vi "oldVisionToGame.vi"(8 "error in (no error)":errorcluster, 10 "Frame and Field Size in":T5 {"Detection Frame Out"."robots_blue"."height" format="%+4.3f"; "Detection Frame Out"."robots_blue"."pixel_y" format="%+4.3f"; "Detection Frame Out"."robots_blue"."pixel_x" format="%+4.3f"; "Detection Frame Out"."robots_blue"."orientation" format="%+4.3f"; "Detection Frame Out"."robots_blue"."y" format="%+4.3f"; "Detection Frame Out"."robots_blue"."confidence" format="%4.3f"; "Detection Frame Out"."robots_blue"."x" format="%+4.3f"; "Detection Frame Out"."robots_yellow"."height" format="%+4.3f"; "Detection Frame Out"."robots_yellow"."pixel_y" format="%+4.3f"; "Detection Frame Out"."robots_yellow"."pixel_x" format="%+4.3f"; "Detection Frame Out"."robots_yellow"."orientation" format="%+4.3f"; "Detection Frame Out"."robots_yellow"."y" format="%+4.3f"; "Detection Frame Out"."robots_yellow"."confidence" format="%4.3f"; "Detection Frame Out"."robots_yellow"."x" format="%+4.3f"}, 11 "Vision in":refnum<class "Vision.lvclass">) -> (0 "error out":errorcluster, 2 "Detection Frame Out":T1 {"robots_blue"."height" format="%+4.3f"; "robots_blue"."pixel_y" format="%+4.3f"; "robots_blue"."pixel_x" format="%+4.3f"; "robots_blue"."orientation" format="%+4.3f"; "robots_blue"."y" format="%+4.3f"; "robots_blue"."confidence" format="%4.3f"; "robots_blue"."x" format="%+4.3f"; "robots_yellow"."height" format="%+4.3f"; "robots_yellow"."pixel_y" format="%+4.3f"; "robots_yellow"."pixel_x" format="%+4.3f"; "robots_yellow"."orientation" format="%+4.3f"; "robots_yellow"."y" format="%+4.3f"; "robots_yellow"."confidence" format="%4.3f"; "robots_yellow"."x" format="%+4.3f"}, 3 "Vision out":refnum<class "Vision.lvclass">)   [LabVIEW 2022 SP3, in "Vision.lvclass"]
uses:
  Vision.lvclass
  Old vision/Controls/SSL Field State.ctl
  Old vision/Controls/SSL Detection Frame.ctl
  Old vision/Controls/SSL Detection Robot.ctl
  <vilib>/Analysis/Matrix/Datatypes/RealMatrix.ctl
  Old vision/Controls/SSL Detection Ball.ctl
  <vilib>/Analysis/Matrix/NI_Matrix.lvlib
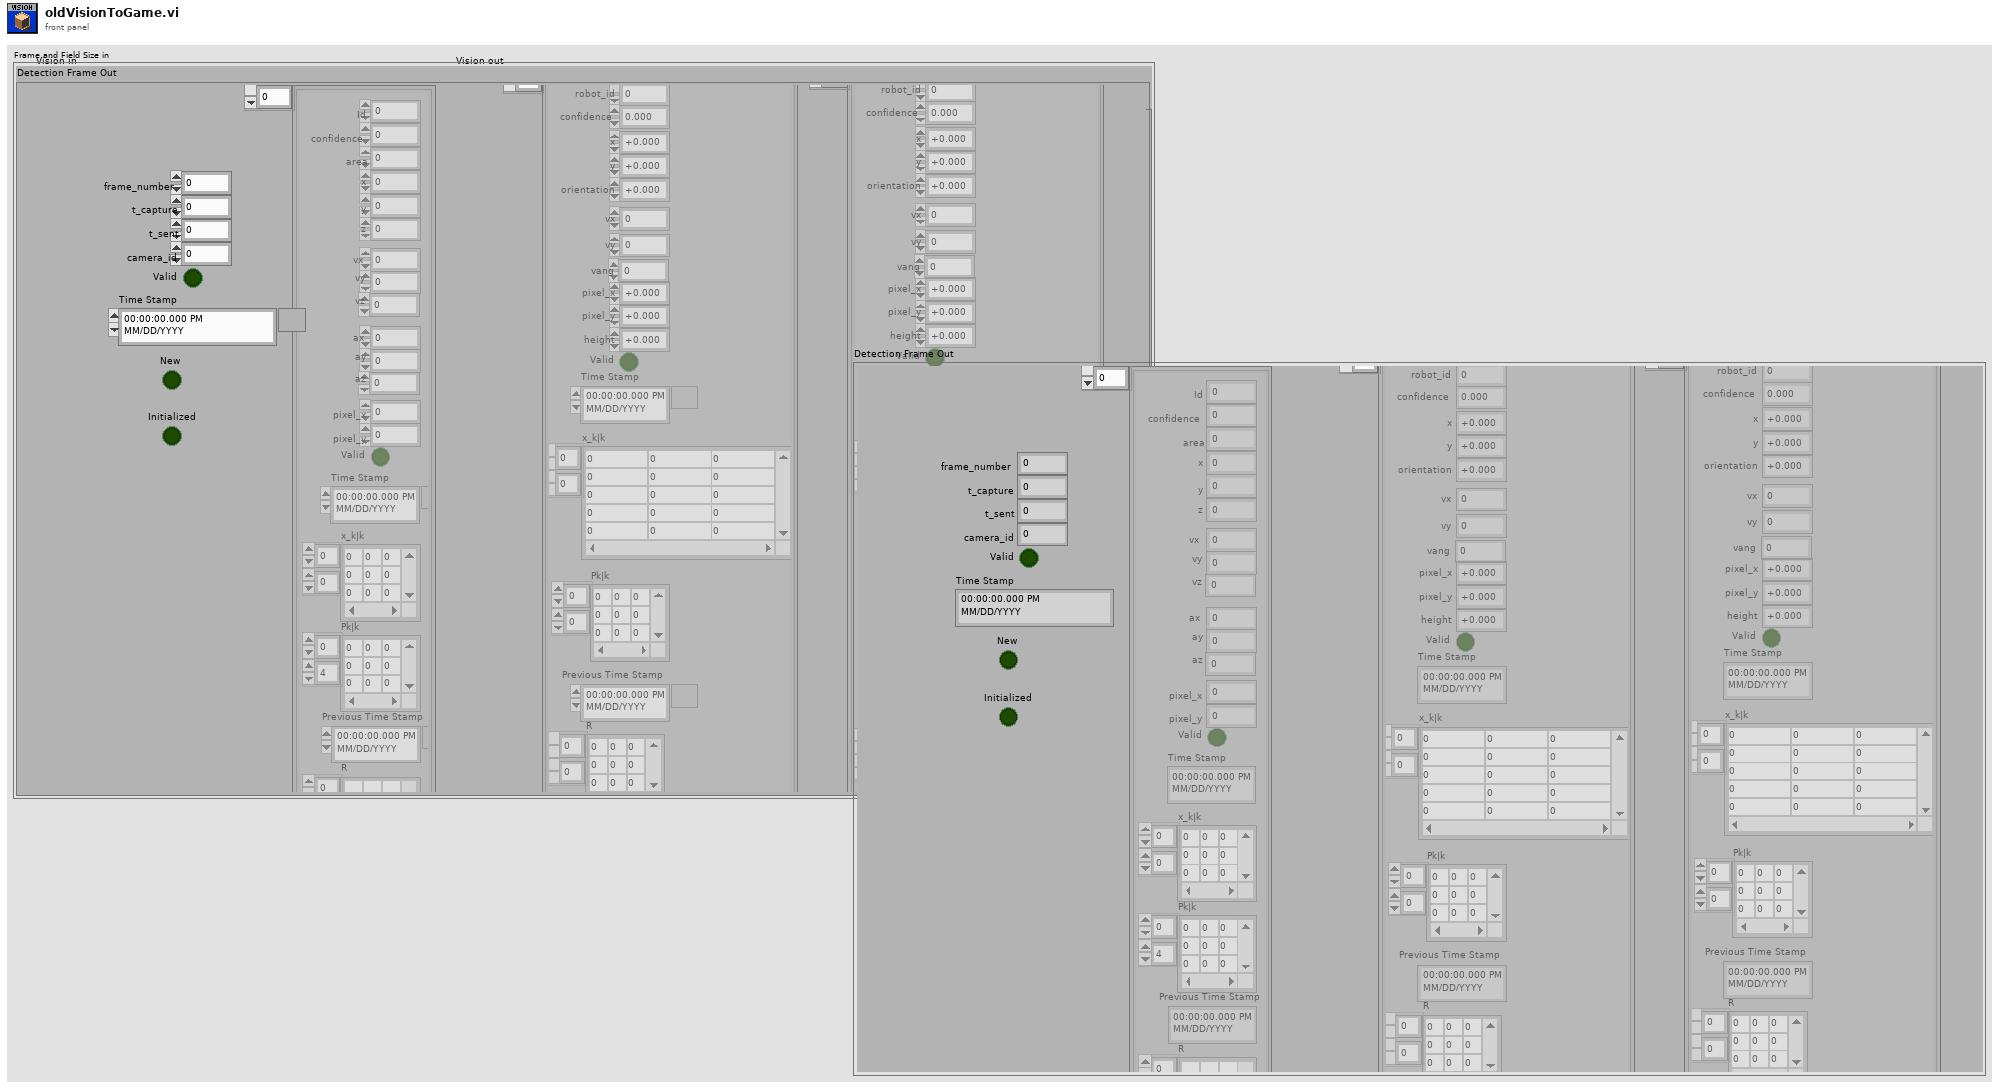
[diagram p1: front panel]
types:
  T1 = typedef "SSL Detection Frame.ctl" = cluster{"frame_number":u32, "t_capture":dbl, "t_sent":dbl, "camera_id":u32, "robots_yellow":T2[], "robots_blue":T2[], "balls":T4[], "Valid":bool, "Time Stamp":timestamp, "New":bool, "Initialized":bool}
  T2 = typedef "SSL Detection Robot.ctl" = cluster{"x":sgl, "robot_id":u32, "confidence":sgl, "y":sgl, "orientation":sgl, "pixel_x":sgl, "pixel_y":sgl, "height":sgl, "Valid":bool, "Time Stamp":timestamp, "x_k|k":T3, "Pk|k":T3, "Previous Time Stamp":timestamp, "R":T3, "vx":dbl, "vy":dbl, "vang":dbl}
  T3 = typedef "NI_Matrix.lvlib/RealMatrix.ctl" = dbl[][]
  T4 = typedef "SSL Detection Ball.ctl" = cluster{"x":sgl, "area":u32, "confidence":sgl, "y":sgl, "z":sgl, "pixel_x":sgl, "pixel_y":sgl, "Valid":bool, "Time Stamp":timestamp, "x_k|k":T3, "Pk|k":T3, "Id":u32, "Previous Time Stamp":timestamp, "R":T3, " vx":sgl, "vy":dbl, "vz":dbl, " ax":sgl, "ay":dbl, "az":dbl}
  T5 = typedef "SSL Field State.ctl" = cluster{"Detection Frame Out":T1, "Field Size Out":cluster{"line_width":u32, "field_length":u32, "field_width":u32, "boundary_width":u32, "referee_width":u32, "goal_width":u32, "goal_depth":u32, "goal_wall_width":u32, "center_circle_radius":u32, "defense_radius":u32, "defense_stretch":u32, "free_kick_from_defense_dist":u32, "penalty_spot_from_field_line_dist":u32, "penalty_line_from_spot_dist":u32}, "Received Time Stamp":timestamp}
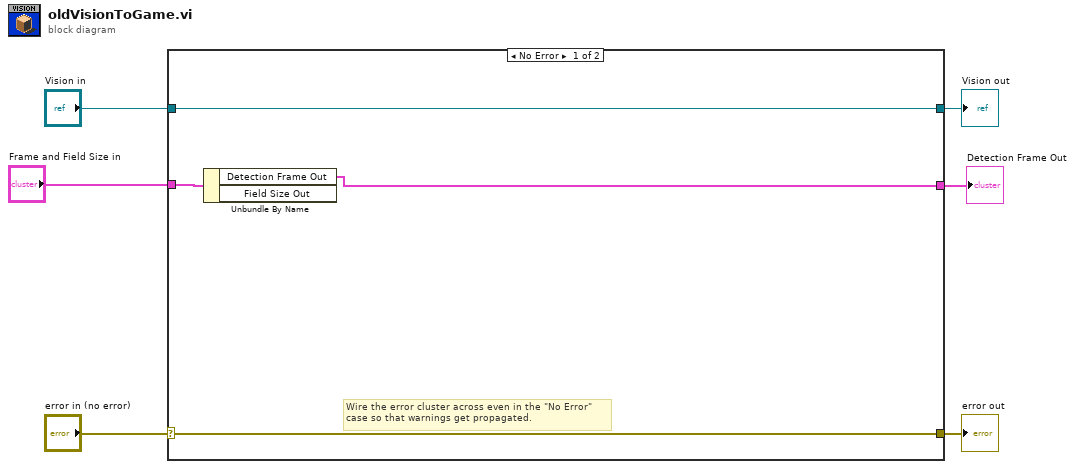
[diagram p0: block diagram]
diagram:
  n1 = case shown="No Error" "error in (no error)" {
    selector: "error in (no error)" -> [w9 w12]
    tunnel: [w9 w12] -> w5
    tunnel: [w10 w11] -> w3
    tunnel: "Vision in" -> [w10 w11]
    tunnel: "Frame and Field Size in" -> [w8 _]
    tunnel: [w7 _] -> w1
    frame No Error {
      # "Wire the error cluster across even in the \"No Error\"\ncase so that warnings get propagated."
      n2 = Unbundle By Name(w8) -> ("Detection Frame Out"=w7:T1)  [unwired: 1 out]
    }
    frame Error {
    }
  }
  "error out" <- w5
  "Vision out" <- w3
  "Detection Frame Out" <- w1
